vi "displayLabels.vi"(8 "error in (no error)":errorcluster, 11 "ActionEditor in":refnum<class "ActionEditor.lvclass">) -> (0 "error out":errorcluster, 3 "ActionEditor out":refnum<class "ActionEditor.lvclass">)   [LabVIEW 2009, in "Views.lvlib" / "ScriptEditor.lvlib" / "ActionEditor.lvclass"]
uses:
  ActionEditor.lvclass
  Tools/Scripting/ScriptingEvent/ScriptEvents/Delay/Delay.lvclass
  ActionEditor.lvclass/ActionEditor.ctl
  Tools/DatabaseHelpers/DbConnection/DeviceDataBase/deviceDataBase.lvclass
  Tools/Scripting/ScriptingEvent/ScriptEvent.lvclass
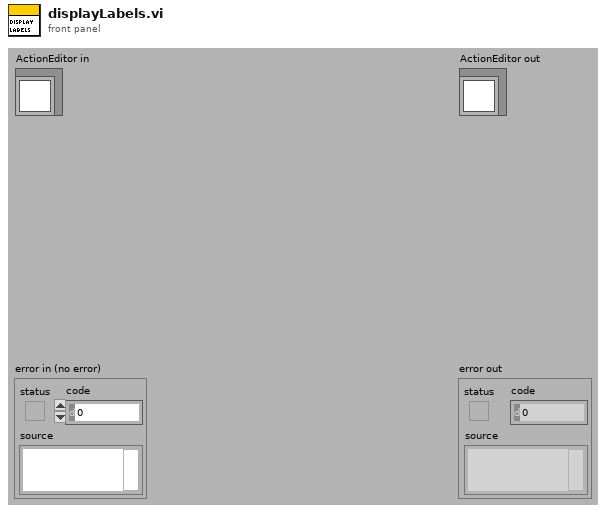
[diagram p1: front panel]
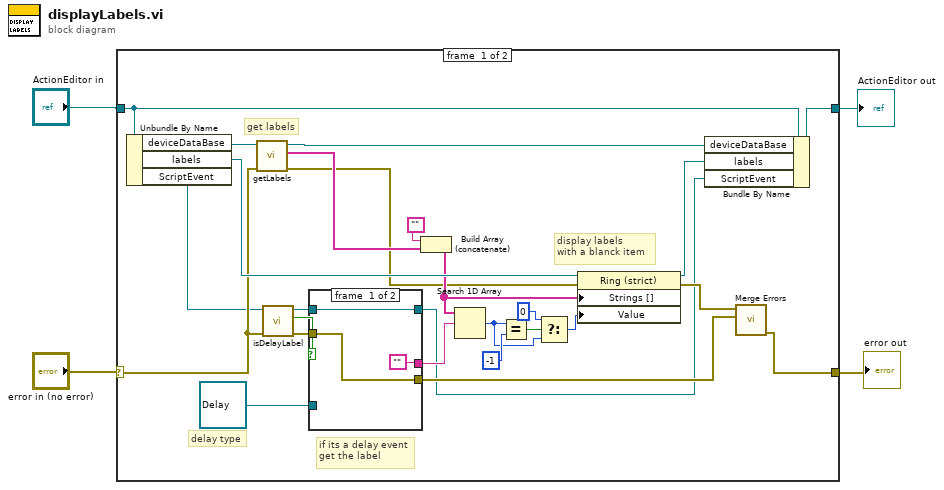
[diagram p0: block diagram]
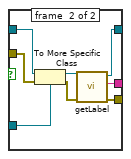
[diagram p2: hidden frame]
diagram:
  n1 = case shown="No Error" "error in (no error)" {
    selector: "error in (no error)" -> [w13 w43]
    tunnel: [w18 w43] -> w1
    tunnel: [w27 w42] -> w2
    tunnel: "ActionEditor in" -> [w28 w42]
    frame #0 {
      # "delay type"
      # "if its a delay event\nget the label"
      # "display labels\nwith a blanck item"
      # "get labels"
      n2 = Unbundle By Name(w28) -> ("deviceDataBase"=w17:refnum<class "deviceDataBase.lvclass">, "labels"=w30:refnum<vi>, "ScriptEvent"=w12:refnum<class "ScriptEvent.lvclass">)
      n3 = call "getLabels.vi"("error in (no error)"=w13, "deviceDataBase in"=w17) -> ("error out"=w14:errorcluster, "labels"=w15:string[], "deviceDataBase out"=w16:refnum<class "deviceDataBase.lvclass">)  [unwired: 7 in]
      n4 = call "isDelayLabel.vi"("error in (no error)"=w13, "ScriptEvent in"=w12) -> ("error out"=w10:errorcluster, "delay"=w11:bool, "ScriptEvent out"=w9:refnum<class "ScriptEvent.lvclass">)  [unwired: 7 in]
      n5 = case shown="False" w11 {
        tunnel: w10 -> [w31 w41]
        tunnel: w9 -> [w32 w40]
        tunnel: refnum<class "Delay.lvclass"> refnum ("Tools.lvlib:Scripting.lvlib:Delay.lvclass") -> [_ w39]
        tunnel: ["" w36] -> w7
        tunnel: [w32 w35] -> w5
        tunnel: [w31 w34] -> w6
        frame #0 {
        }
        frame #1 {
          n6 = To More Specific Class(target class=w39, reference=w40, error in=w41) -> (specific class reference=w38:refnum<class "Delay.lvclass">, error out=w37:errorcluster)
          n7 = call "getLabel.vi"("error in (no error)"=w37, "Delay in"=w38) -> ("error out"=w34:errorcluster, "label"=w36:string, "Delay out"=w35:refnum<class "Delay.lvclass">)  [unwired: 7 in]
        }
      }
      n8 = Build Array (concatenate)("", w15) -> (w25:string[])
      n9 = Search 1D Array(1D array=w25, element=w7) -> (index of element=w21:i32)  [unwired: 1 in]
      n10 = Equal?(x=w21, y=-1) -> (x = y?=w23:bool)
      n11 = Select(t=0, s=w23, f=w21) -> (s? t:f=w20:i32)
      n12 = property class="Ring (strict)"(reference=w30, error in=w14, "Strings []"=w25, "Value"=w20) -> (reference out=w29:refnum<vi>, error out=w19:errorcluster)
      n13 = Bundle By Name(cluster=w28, "deviceDataBase"=w16, "labels"=w29, "ScriptEvent"=w5) -> (w27:refnum<class "ActionEditor.lvclass">)
      n14 = call <vilib>:"Merge Errors.vi"("error in 2 (no error)"=w6, "error in 1 (no error)"=w19) -> ("error out"=w18:errorcluster)  [unwired: 5 in]
    }
    frame #1 {
    }
  }
  "error out" <- w1
  "ActionEditor out" <- w2
